vi "LM Cubic Spline + Sine and gradient.vi"(3 "output control":T1, 4 "data":variant, 5 "X":dbl[](array[numeric]), 6 "a":dbl[](array[numeric])) -> (0 "error out":errorcluster, 1 "f'(X,a)":dbl[][](array[numeric]), 2 "f(X,a)":dbl[](array[numeric]))   [LabVIEW 2021, in "Fits.lvlib"]
doc: "This template is the starting point for creating a model function to be passed to the Nonlinear Curve Fit.vi."
uses:
  Fits.lvlib
  <vilib>/gmath/NumericalOptimization/LM_output select.ctl
  Cubic Spline + Sine Options.ctl
  <vilib>/Analysis/baseanly.llb/Matrix Type of Inverse Matrix.ctl
  <vilib>/Utility/error.llb/DialogType.ctl
  <vilib>/Analysis/baseanly.llb/A x Vector.vi
  <vilib>/Analysis/7linalg.llb/Solve Linear Equations (single right hand).vi
  <vilib>/Analysis/baseanly.llb/Solve Linear Equations By Cholesky.vi
  <vilib>/Analysis/baseanly.llb/Real Matrix to Compact Array.vi
  <vilib>/Analysis/baseanly.llb/Real Compact Tri-Matrix Linear Eqs.vi
  <vilib>/Analysis/7linalg.llb/Solve Linear Eqs (General).vi
  <vilib>/Analysis/7linalg.llb/Solve Linear Eqs (Gen, single right hand).vi
  <vilib>/Analysis/NI_AALPro.lvlib
  <vilib>/Analysis/NI_AALBase.lvlib
  33e4ae97-e3ad-4bc5-842b-10e2724d40c6.vi
  e3cdb349-c702-4513-9d3e-00cb5bd1d2d1.vi
  <vilib>/gmath/NI_Gmath.lvlib
panel:
  # "Parameters:\n\n{y_i}, {a_i}"
  # "Data:\n\nn, T, t_0"
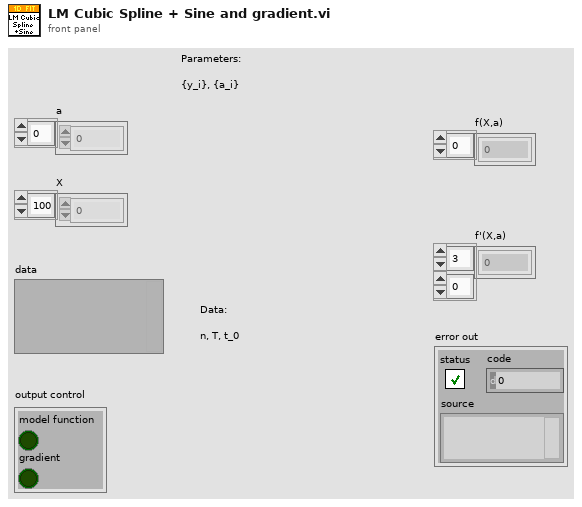
[diagram p1: front panel]
types:
  T1 = typedef "NI_Gmath.lvlib/LM_output select.ctl" = cluster{"model function":bool, "gradient":bool}
  T2 = typedef "Fits.lvlib/Cubic Spline + Sine Options.ctl" = cluster{"Truncation Order":i32, "Period":dbl, "Offset":dbl}
  T3 = typedef "Real Matrix NI_Silver.ctl" = dbl[][]
  T4 = typedef "NI_AALBase.lvlib/Matrix Type of Inverse Matrix.ctl" = enum32{"General", "Positive Definite", "Lower Triangular", "Upper Triangular"}
  T5 = typedef "DialogType.ctl" = u16
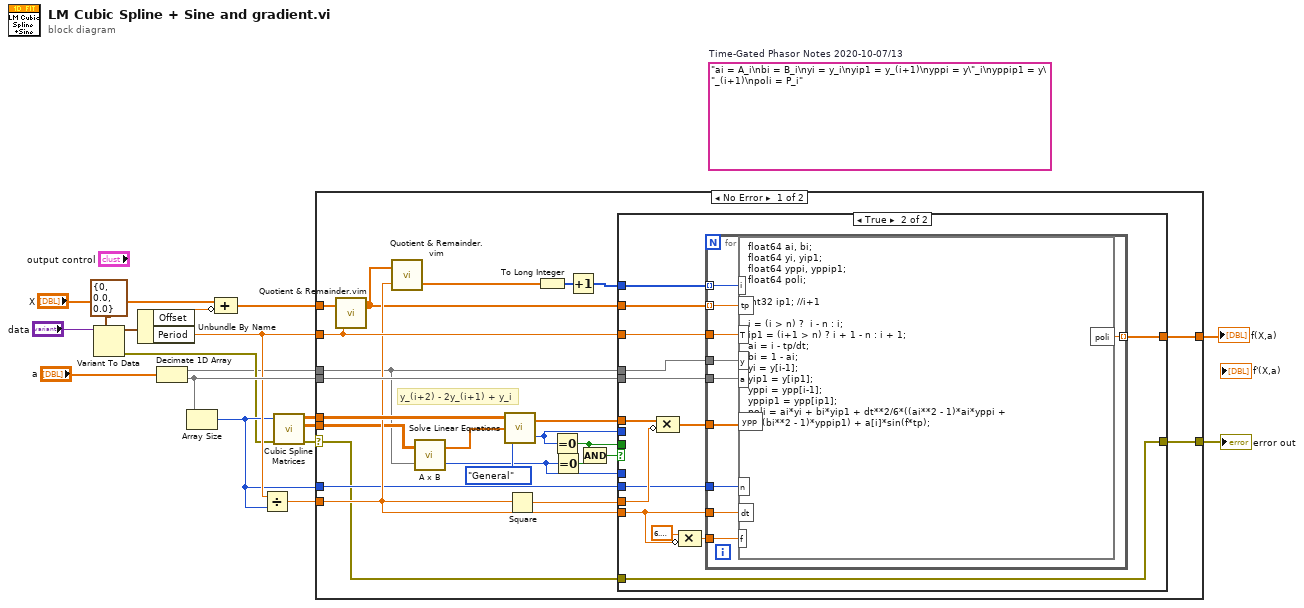
[diagram p0: block diagram]
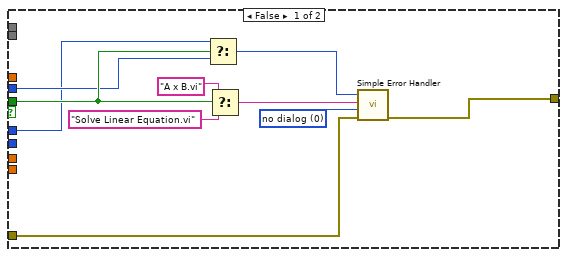
[diagram p2: hidden frame]
diagram:
  (unwired) "ai = A_i\nbi = B_i\nyi = y_i\nyip1 = y_(i+1)\nyppi = y\"_i\nyppip1 = y\"_(i+1)\npoli = P_i"  # Time-Gated Phasor Notes 2020-10-07/13
  n1 = Variant To Data(type=T2 {"Truncation Order"=0, "Period"=0.0, "Offset"=0.0} ("Cubic Spline + Sine Options"), Variant="data") -> (data=w15:T2, error out=w7:errorcluster)  [unwired: 1 in]
  n2 = Unbundle By Name(w15) -> ("Offset"=w3:dbl, "Period"=w11:dbl)
  n3 = Decimate 1D Array("a") -> (w2:dbl[], w14:dbl[])
  n4 = Array Size(array=w14) -> (size(s)=w9:i32)
  n5 = Compound Arithmetic op=ADD("X", invert w3) -> (w12:dbl[])
  n6 = Divide(x=w11, y=w9) -> (x/y=w10:dbl)
  n7 = call "Cubic Spline Matrices.vi"("Error In"=w7, "order"=w9) -> ("Error Out"=w8:errorcluster, "Cubic Spline nxn Matrix Q"=w1:T3, "Cubic Spline nxn Matrix M"=w13:T3)  [unwired: 7 in]
  n8 = case shown="No Error" w8 {
    selector: w8 -> [w30 w77]
    tunnel: [w42 _] -> w18
    tunnel: w14 -> [w41 _]
    tunnel: w13 -> [w40 _]
    tunnel: w2 -> [w27 _]
    tunnel: w12 -> [w36 _]
    tunnel: w11 -> [w35 _]
    tunnel: w10 -> [w32 _]
    tunnel: w9 -> [w31 _]
    tunnel: [w29 w77] -> w6
    tunnel: w1 -> [w28 _]
    frame No Error {
      # "y_(i+2) - 2y_(i+1) + y_i"
      n9 = call "Quotient & Remainder.vim"("y"=w35, "x"=w36) -> ("x - E(x/y)y"=w25:dbl[])  [unwired: 1 out]
      n10 = call "Quotient & Remainder.vim"("y"=w32, "x"=w25) -> ("E(x/y)"=w34:dbl[])  [unwired: 1 out]
      n11 = call-poly <vilib>:"A x B.vi"("Vector"=w27, "A"=w28) -> ("error"=w20:i32, "A x Vector"=w26:dbl[])
      n12 = call-poly <vilib>:"Solve Linear Equations.vi"("matrix type"=Matrix_Type_of_Inverse_Matrix."General", "Known Vector"=w26, "Input Matrix"=w40) -> ("error"=w19:i32, "Solution Vector"=w39:dbl[])
      n13 = Square(x=w32) -> (x^2=w37:dbl)
      n14 = To Long Integer(number=w34) -> (32bit integer=w24:i32[])
      n15 = Equal To 0?(x=w19) -> (x = 0?=w21:bool)
      n16 = Equal To 0?(x=w20) -> (x = 0?=w22:bool)
      n17 = Increment(x=w24) -> (x+1=w33:i32[])
      n18 = Compound Arithmetic op=AND(w21, w22) -> (w23:bool)
      n19 = case shown="True" w23 {
        tunnel: [_ w66] -> w42
        tunnel: w41 -> [_ w65]
        tunnel: w27 -> [_ w64]
        tunnel: w39 -> [_ w63]
        tunnel: w37 -> [_ w61]
        tunnel: w35 -> [_ w60]
        tunnel: w33 -> [_ w59]
        tunnel: w25 -> [_ w58]
        tunnel: w32 -> [_ w57]
        tunnel: w31 -> [_ w54]
        tunnel: w30 -> [w52 w53]
        tunnel: [w51 w53] -> w29
        tunnel: w21 -> [w46 _]
        tunnel: w20 -> [w44 _]
        tunnel: w19 -> [w45 _]
        frame False {
          w50 = T5 0 items=["no dialog", "OK message", "continue or stop message", "OK message + warnings", "continue/stop + warnings"] ("type of dialog (OK msg:1)")
          n20 = Select(t=w44, s=w46, f=w45) -> (s? t:f=w43:i32)
          n21 = Select(t="A x B.vi" ("error source (\" \")"), s=w46, f="Solve Linear Equation.vi" ("error source (\" \")")) -> (s? t:f=w47:string)
          n22 = call <vilib>:"Simple Error Handler.vi"("error code (no error:0)"=w43, "error source (\" \")"=w47, "type of dialog (OK msg:1)"=w50, "error in (no error)"=w52) -> ("error out"=w51:errorcluster)  [unwired: 1 in, 4 out]
        }
        frame True {
          n23 = Compound Arithmetic op=MULTIPLY(w63, invert w61) -> (w62:dbl[])
          n24 = Compound Arithmetic op=MULTIPLY(6.283185307179586, invert w57) -> (w55:dbl)
          n25 = for {
            tunnel: [w76] -> w66 mode=indexing
            tunnel: w64 -> [w75]
            tunnel: w65 -> [w74]
            tunnel: w58 -> [w73] mode=indexing
            tunnel: w60 -> [w72]
            tunnel: w62 -> [w71]
            tunnel: w59 -> [w70] mode=indexing
            tunnel: w57 -> [w69]
            tunnel: w55 -> [w68]
            tunnel: w54 -> [w67]
            n26 = formula code="float64 ai, bi;\nfloat64 yi, yip1;\nfloat64 yppi, yppip1;\nfloat64 poli;\n\nint32 ip1; //i+1\n\ni = (i > n) ?  i - n : i;\nip1 = (i+1 > n) ? i + 1 - n : i + 1;\nai = i - tp/dt;\nbi = 1 - ai;\nyi = y[i-1];\nyip1 = y[ip1];\nyppi = ypp[i-1];\nyppip1 = ypp[ip1];\npoli = ai*yi + bi*yip1 + dt**2/6*((ai**2 - 1)*ai*yppi + \nbi*(bi**2 - 1)*yppip1) + a[i]*sin(f*tp);"("y"=w75, "a"=w74, "T"=w72, "tp"=w73, "ypp"=w71, "i"=w70, "dt"=w69, "f"=w68, "n"=w67) -> ("poli"=w76:dbl)
          }
        }
      }
    }
    frame Error {
    }
  }
  "f(X,a)" <- w18
  "error out" <- w6
